vi "Execute Dig Grave.vi"(6 "Mouse Position":T1, 8 "User VI Ref":refnum<vi>, 9 "Menu Item Tag Suffix":string, 10 "Remaining Items":refnum<vi>[](array[refnum]), 11 "Affected Items":T2) -> (0 "Fail transaction?":bool)   [LabVIEW 2017, in "Eulogy.lvlib" / "Shortcut Menu.lvlib"]
doc: "This VI is part of a plug-in for modifying the LabVIEW shortcut menus. This is the execute VI which is called when the shortcut menu is chosen by the user. It performs the action of the selected menu item."
uses:
  Shortcut Menu.lvlib
  Dig Grave.ctl
  <vilib>/Utility/miscctls.llb/LVPositionTypeDef.ctl
  Eulogy.lvlib
panel:
  # "All controls on this panel except \"Affected Items\" have been locked to prevent accidental edits. Changing the control names or types, other than the elements of the \"Affected Items\" cluster will make the VI unusable as a menu plugin.\n\nSee Context Help for each control for details about its use."
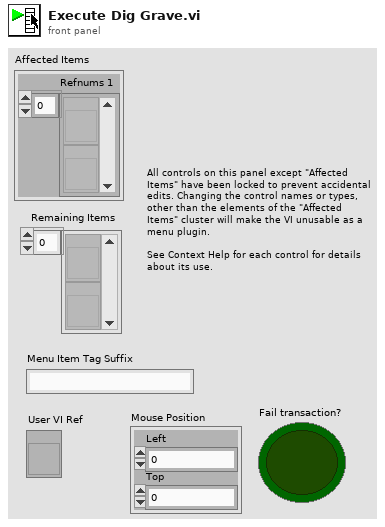
[diagram p1: front panel]
types:
  T1 = typedef "LVPositionTypeDef.ctl" = cluster{"Left":i32, "Top":i32}
  T2 = typedef "Eulogy.lvlib/Shortcut Menu.lvlib/Dig Grave.ctl" = cluster{"Refnums 1":refnum<vi>[]}
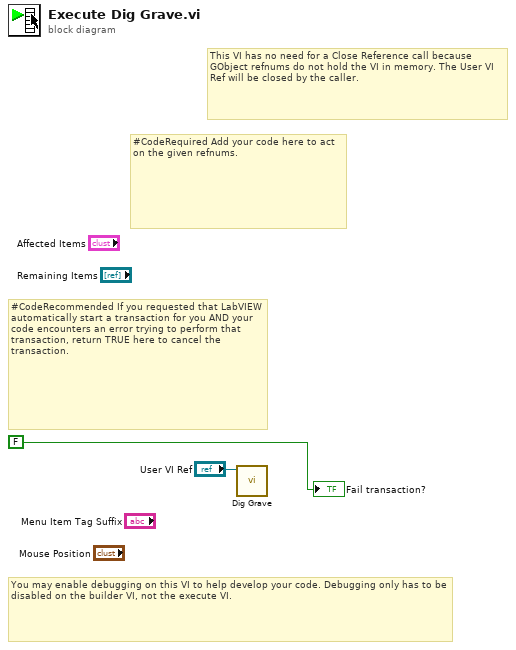
[diagram p0: block diagram]
diagram:
  # "You may enable debugging on this VI to help develop your code. Debugging only has to be disabled on the builder VI, not the execute VI."
  # "#CodeRecommended If you requested that LabVIEW automatically start a transaction for you AND your code encounters an error trying to perform that transaction, return TRUE here to cancel the transaction."
  # "#CodeRequired Add your code here to act on the given refnums."
  # "This VI has no need for a Close Reference call because GObject refnums do not hold the VI in memory. The User VI Ref will be closed by the caller."
  n1 = call "Dig Grave.vi"("VI In"="User VI Ref") -> ()  [unwired: 9 in, 2 out]
  "Fail transaction?" <- FALSE
